vi "User Event FG.vi"(7 "User Event Actions":enum16{"Destroy", "Create", "Get"}(ring), 8 "error in":errorcluster) -> (0 "error out":errorcluster, 3 "Event Item":refnum<user-event>)   [LabVIEW 2015, in "Generic Module Library.lvlib" / "Template G_Module.lvlib"]
uses:
  Template G_Module.lvlib
  Private Controls/Event Item.ctl
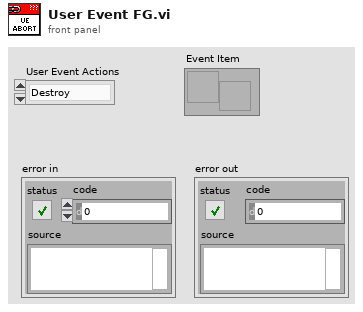
[diagram p1: front panel]
types:
  T1 = typedef "Generic Module Library.lvlib/Template G_Module.lvlib/Event Item.ctl" = cluster{"Event Data":variant}
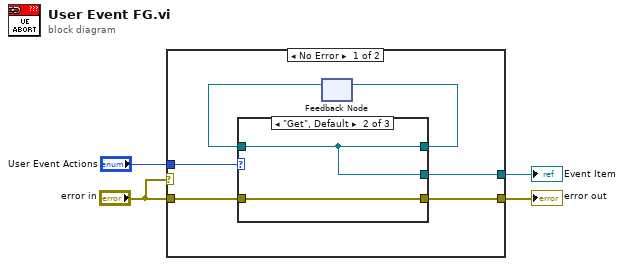
[diagram p0: block diagram]
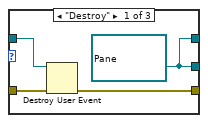
[diagram p2: hidden frame]
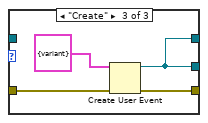
[diagram p3: hidden frame]
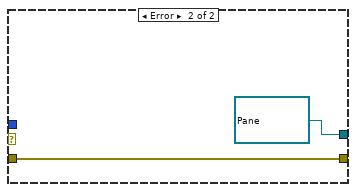
[diagram p4: hidden frame]
diagram:
  n1 = case shown="No Error" "error in" {
    tunnel: "error in" -> [w10 w22]
    tunnel: "User Event Actions" -> [w9 _]
    tunnel: [w8 w22] -> w4
    tunnel: [w6 refnum<user-event> refnum ("Event Item")] -> w1
    frame No Error {
      n2 = feedback #1() -> (w7:refnum<user-event>)  [unwired: 1 in]
      n3 = case shown="\"Get\", Default" w9 {
        tunnel: w10 -> [w14 w16 w20]
        tunnel: [w13 w16 w19] -> w8
        tunnel: w7 -> [w12 w15 _]
        tunnel: [w11 w15 w17] -> w6
        tunnel: [w11 w15 w17] -> w5
        frame "Destroy" {
          w11 = refnum<user-event> refnum ("Event Item")
          n4 = Destroy User Event(user event=w12, error in=w14) -> (error out=w13:errorcluster)
        }
        frame "Get", Default {
        }
        frame "Create" {
          n5 = Create User Event(user event datatype=T1 {"Event Data"=variant} ("Event Item"), error in=w20) -> (user event=w17:refnum<user-event>, error out=w19:errorcluster)
        }
      }
      n6 = feedback-in #1(w5) -> ()
    }
    frame Error {
    }
  }
  "error out" <- w4
  "Event Item" <- w1
